vi "Specified_Channels_client.vi"(6 "Mode":T1, 9 "End time":dbl, 10 "Start time":dbl, 11 "ADAM Index array":i32[](array[numeric])) -> (0 "Output array":dbl[][](array[numeric]) format="%.2f", 1 "Averaging Period":dbl[](array[numeric]) format="%.2f", 2 "Centre Times":dbl[](array[numeric]) format="%.2f", 3 "All Active Ch Names":string[](array[string]), 4 "Messages":string)   [LabVIEW 2010]
doc: "This is an example of using features of the VI Server as a client. It shows how you might browse from one or more applications that may be exporting data from one or more data stations. \n\nThe example shows how to query a server for its list of exported VIs, how to get references to the VIs, and how call them with the Call By Reference function."
uses:
  Sub VIs/ADAM Controls/Search_mode.ctl
  Anemometry/Anemometry Sub Vis/Controls/Server_Comms.ctl
  Anemometry/Anemometry Sub Vis/Globals/Preference_global.vi
panel:
  in  "vi type":refnum<vi>
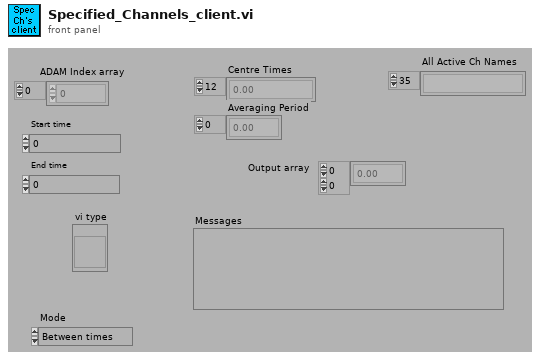
[diagram p1: front panel]
types:
  T1 = typedef "Search_mode.ctl" = enum16{"Between times", "All Times"}
  T2 = typedef "Server_Comms.ctl" = enum16{"Server Link Healthy", "Do Not Link To Server"}
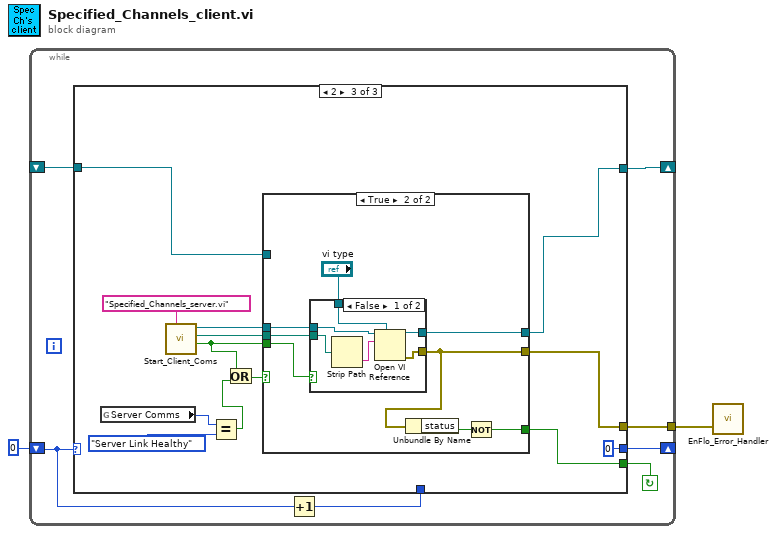
[diagram p0: block diagram]
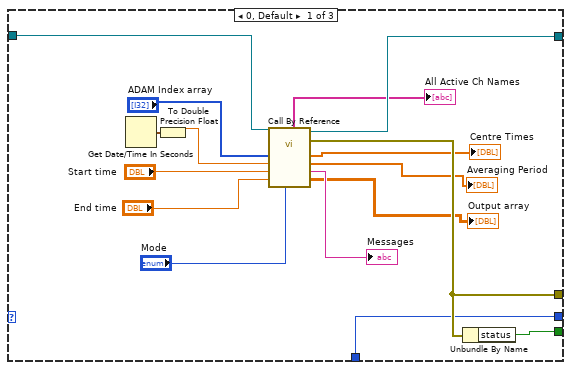
[diagram p2: hidden frame]
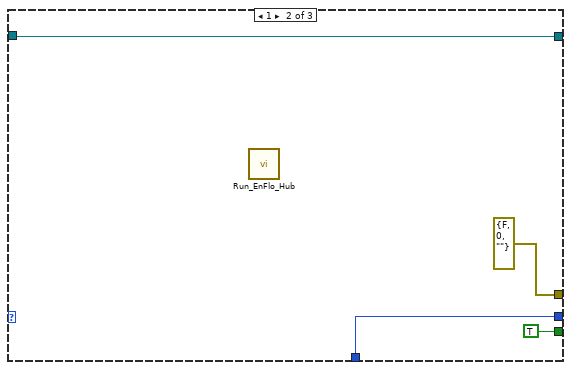
[diagram p3: hidden frame]
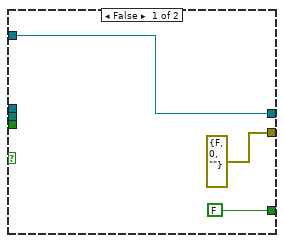
[diagram p4: hidden frame]
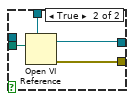
[diagram p5: hidden frame]
diagram:
  n1 = while {
    shift-left: 0 -> [w3]
    shift-right: [w5] -> _
    tunnel: [w7] -> w2
    shift-left: _ -> [w6]
    shift-right: [w9] -> _
    stop <- w8 continue-if-true
    n2 = Increment(x=w3) -> (x+1=w4:i32)
    n3 = case shown="2" w3 {
      tunnel: [w19 w29 w42] -> w9
      tunnel: [w17 TRUE ("status") w31] -> w8
      tunnel: [w18 errorcluster {"status"=FALSE, "code"=0, "source"=""} w41] -> w7
      tunnel: w6 -> [w21 w29 w32]
      tunnel: [w11 w28 0] -> w5
      tunnel: w4 -> [w11 w28 _]
      frame 0, Default {
        n4 = Get Date/Time In Seconds() -> (seconds since 1Jan1904=w10:timestamp)
        n5 = To Double Precision Float(number=w10) -> (double precision float=w20:dbl)
        n6 = call-by-ref "?"(reference=w21, "Mode"="Mode", "End time"="End time", "Start time"="Start time", "Clients time"=w20, "Requested channels"="ADAM Index array") -> (reference out=w19:refnum<vi>, error out=w18:errorcluster, "Output array"=→"Output array":dbl[][], "Messages"=→"Messages":string, "Averaging Period"=→"Averaging Period":dbl[], "Centre Times"=→"Centre Times":dbl[], "All Active Ch Names"=→"All Active Ch Names":string[])  [unwired: 1 in]
        n7 = Unbundle By Name(w18) -> ("status"=w17:bool)
      }
      frame 1 {
        n8 = call "Run_EnFlo_Hub.vi"() -> ()  [unwired: 8 out]
      }
      frame 2 {
        n9 = global read "Preference_global.vi" "Server Comms"() -> (w36:T2)
        n10 = call "Start_Client_Coms.vi"("VI name to run on server"="Specified_Channels_server.vi") -> ("LabVIEW application reference"=w38:refnum<vi>, "Checked VI name"=w39:path, "Local Call"=w34:bool)  [unwired: 1 in, 1 out]
        n11 = Equal?(x=w36, y=Server_Comms."Server Link Healthy" ("Server Comms")) -> (x = y?=w35:bool)
        n12 = Or(x=w34, y=w35) -> (x .or. y?=w33:bool)
        n13 = case shown="True" w33 {
          tunnel: [w44 w53] -> w42
          tunnel: [errorcluster {"status"=FALSE, "code"=0, "source"=""} ("error out") w48] -> w41
          tunnel: w39 -> [_ w52]
          tunnel: w38 -> [_ w51]
          tunnel: w34 -> [_ w50]
          tunnel: w32 -> [w44 _]
          tunnel: [FALSE ("status") w46] -> w31
          frame False {
          }
          frame True {
            n14 = case shown="False" w50 {
              tunnel: [w58 w63] -> w53
              tunnel: "vi type" -> [w55 w62]
              tunnel: w52 -> [w56 w61]
              tunnel: w51 -> [w54 _]
              tunnel: [w57 w60] -> w48
              frame False {
                n15 = Strip Path(path=w56) -> (name=w59:string)  [unwired: 1 out]
                n16 = Open VI Reference(type specifier VI Refnum (for type only)=w55, application reference (local)=w54, vi path=w59) -> (vi reference=w58:refnum<vi>, error out=w57:errorcluster)  [unwired: 1 in, 2 out]
              }
              frame True {
                n17 = Open VI Reference(type specifier VI Refnum (for type only)=w62, vi path=w61) -> (vi reference=w63:refnum<vi>, error out=w60:errorcluster)  [unwired: 1 in, 3 out]
              }
            }
            n18 = Unbundle By Name(w48) -> ("status"=w47:bool)
            n19 = Not(x=w47) -> (.not. x?=w46:bool)
          }
        }
      }
    }
  }
  n20 = call "EnFlo_Error_Handler.vi"("error in (no error)"=w2) -> ()  [unwired: 2 in, 3 out]
